vi "Do.vi"(8 "error in (no error)":errorcluster, 10 "Actor in":refnum<class "Actor.lvclass">, 11 "Enable Process Alarm Logging Msg":refnum<class "Enable Process Alarm Logging Msg.lvclass">) -> (0 "error out":errorcluster, 2 "Actor out":refnum<class "Actor.lvclass">)   [LabVIEW 2016, in "CS++DSCManager.lvlib" / "Enable Process Alarm Logging Msg.lvclass"]
doc: "This VI delivers the message to the actor by calling the appropriate method(s) on the actor."
uses:
  Enable Process Alarm Logging Msg.lvclass
  <vilib>/ActorFramework/Actor/Actor.lvclass
  CS++DSCManager/CS++DSCManager.lvclass
  C:/Program Files (x86)/National Instruments/LabVIEW 2016/vi.lib/ActorFramework/Actor/Actor.lvclass
  Enable Process Alarm Logging Msg.lvclass/Enable Process Alarm Logging Msg.ctl
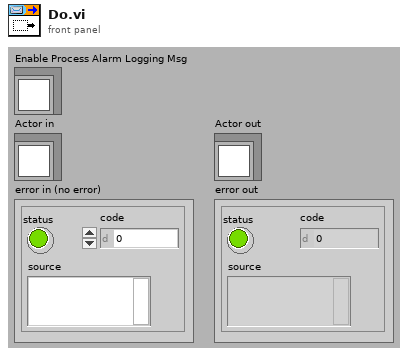
[diagram p1: front panel]
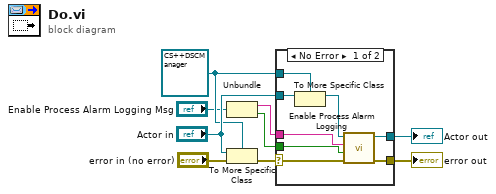
[diagram p0: block diagram]
diagram:
  w4 = refnum<class "CS++DSCManager.lvclass"> refnum ("Actor in")
  n1 = Unbundle ("Main-Unbundle")("Enable Process Alarm Logging Msg") -> (w2:string, w1:bool)
  n2 = To More Specific Class(target class=w4, reference="Actor in", error in="error in (no error)") -> (error out=w8:errorcluster)  [unwired: 1 out]
  n3 = case shown="No Error" w8 {
    selector: w8 -> [w15 w19]
    tunnel: [w17 w19] -> w7
    tunnel: [w16 w18] -> w6
    tunnel: "Actor in" -> [w14 w18]
    tunnel: w4 -> [w13 _]
    tunnel: w2 -> [w11 _]
    tunnel: w1 -> [w10 _]
    frame No Error {
      n4 = To More Specific Class(target class=w13, reference=w14) -> (specific class reference=w12:refnum<class "CS++DSCManager.lvclass">)  [unwired: 1 in, 1 out]
      n5 = call "Enable Process Alarm Logging.vi"("Error In"=w15, "Log?"=w10, "Process Name"=w11, "CS++DSCManager in"=w12) -> ("Error Out"=w17:errorcluster, "CS++DSCManager out"=w16:refnum<class "CS++DSCManager.lvclass">)  [unwired: 6 in]
    }
    frame Error {
    }
  }
  "error out" <- w7
  "Actor out" <- w6
